vi "calibrate RP.vi"() -> ()   [LabVIEW 2018]
uses:
  Libraries/Instruments/Pulse Driver/Pusle Driver Configuration.ctl
  Libraries/Red Pitaya/RP EEPROM Calibration.ctl
  Libraries/Red Pitaya/Red Pitaya Digitizer/Red Pitaya Digitizer.lvclass
  C:/github/NHMFL_Core/Libraries/Instruments/Pulse Driver/Pulse Driver.lvclass
  Libraries/Red Pitaya/Red Pitaya Digitizer/Red Pitaya Digitizer.lvclass/Red Pitaya Digitizer.ctl
  Libraries/Red Pitaya/Red Pitaya Digitizer/Read RP Instrument.vi
  Libraries/Red Pitaya/Red Pitaya Digitizer/Write Server address.vi
  Libraries/Red Pitaya/RP Core/RP Instrument/RP Instrument.lvclass
panel:
  out "return code":i32
  out "Server  output":string
  in  "Write calib":bool
  in  "calib parameters":string
  in  "Read calib":bool
  out "Ch1 Mean (DC)":dbl
  out "Ch1 Peak to Peak":dbl
  out "Ch2 Mean (DC)":dbl
  out "Ch1 Peak to Peak":dbl
  out "RP EEPROM Calibration":T1 {"magic" format="%x"}
  in  "milliseconds to wait":u32
  out "Waveform Graph":i16[][](graph)
  in  "Server address":string="192.168.1.100"
  in  "Pulse Configuration":T2={"Pre-trigger duration"=0.01, "Post-trigger duration"=0.1, "Rate"=1000000.0, "Ranges"=[10.0], "Re-name channels"=[], "Active channels"="0:1", "External clock"=FALSE} {"Rate" format="%#_8pHz"; "Post-trigger duration" format="%#_6ps"; "Pre-trigger duration" format="%#_6ps"; "Ranges" format="%#_6pV"}
  in  "Read data":bool
  in  "stop":bool
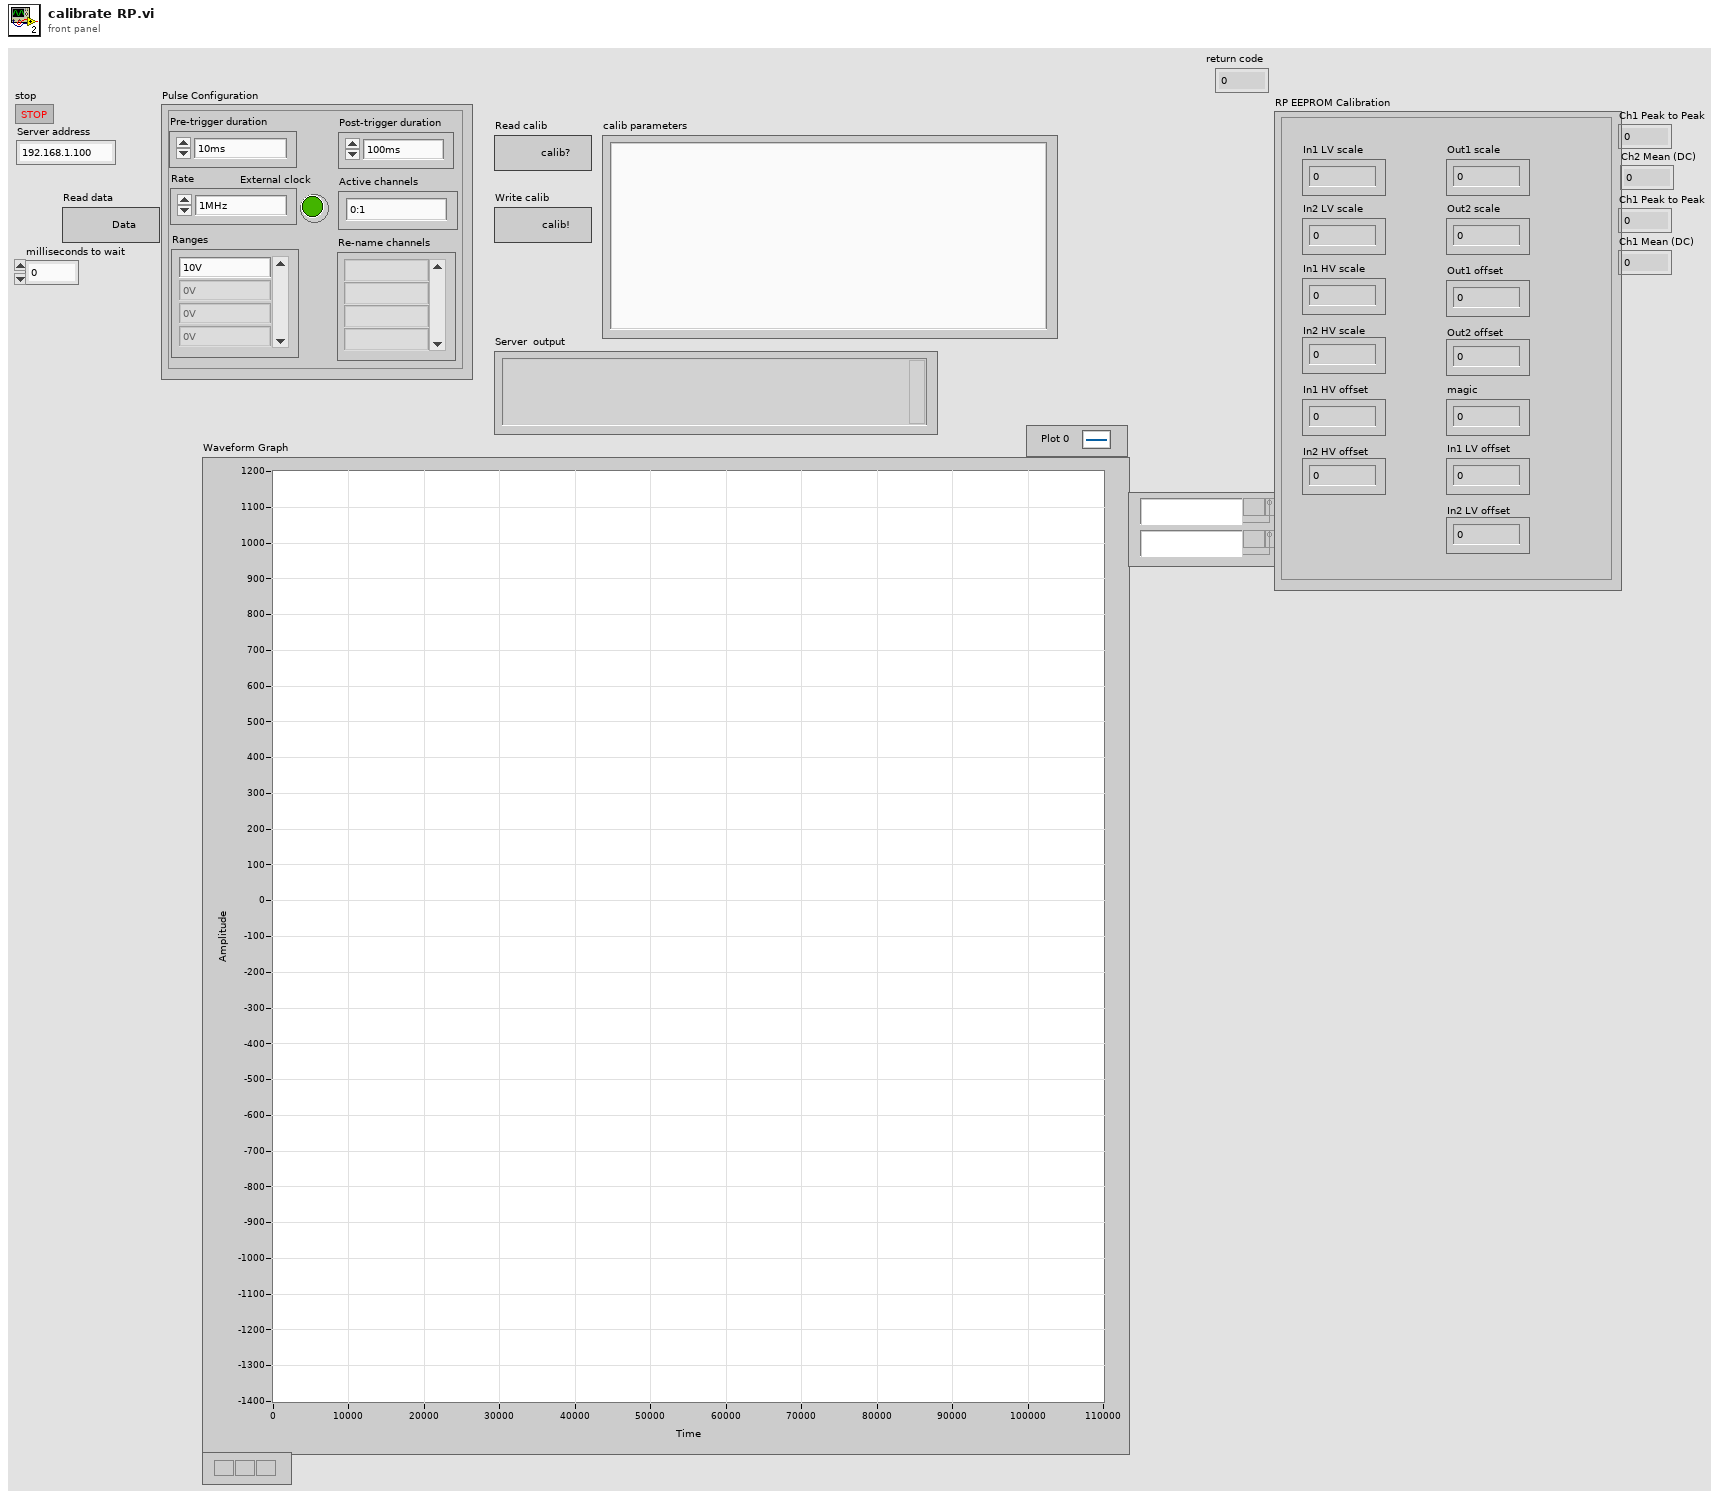
[diagram p1: front panel]
types:
  T1 = typedef "RP EEPROM Calibration.ctl" = cluster{"In1 LV scale":u32, "In2 LV scale":u32, "In1 HV scale":u32, "In2 HV scale":u32, "In1 HV offset":i32, "In2 HV offset":i32, "Out1 scale":u32, "Out2 scale":u32, "Out1 offset":i32, "Out2 offset":i32, "magic":u32, "In1 LV offset":i32, "In2 LV offset":i32}
  T2 = typedef "Pusle Driver Configuration.ctl" = cluster{"Pre-trigger duration":dbl, "Post-trigger duration":dbl, "Rate":dbl, "Ranges":dbl[], "Re-name channels":string[], "Active channels":string, "External clock":bool}
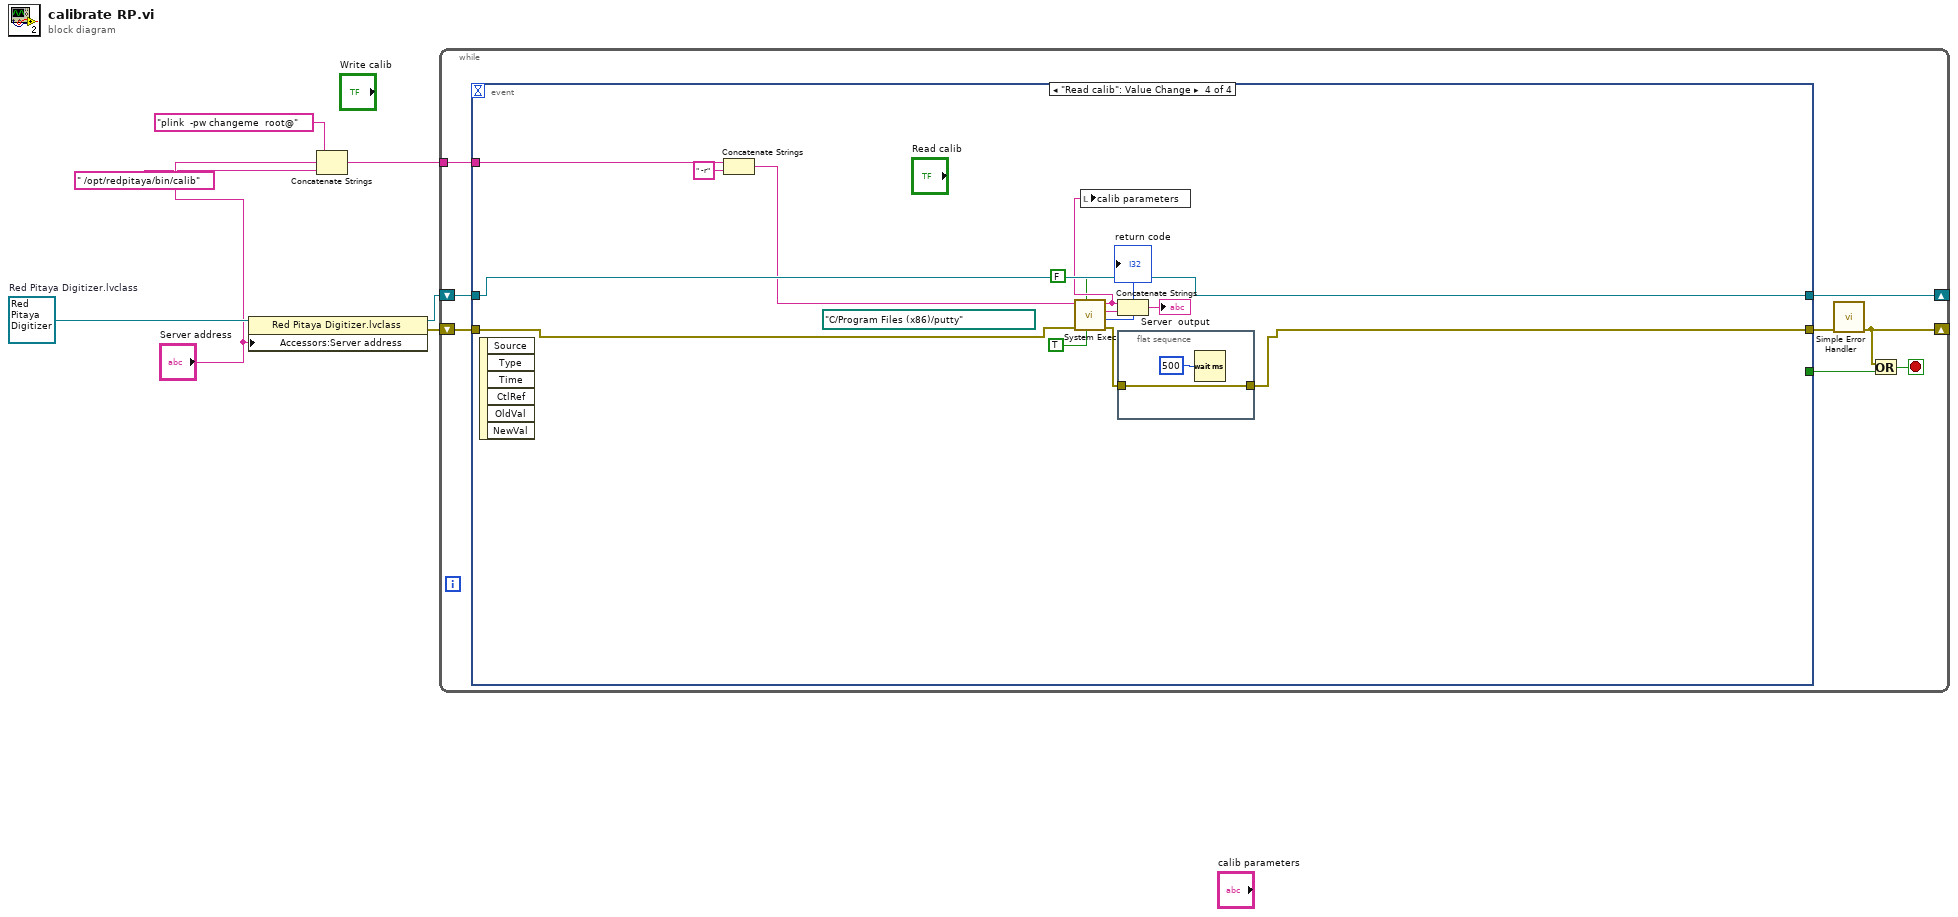
[diagram p0: block diagram]
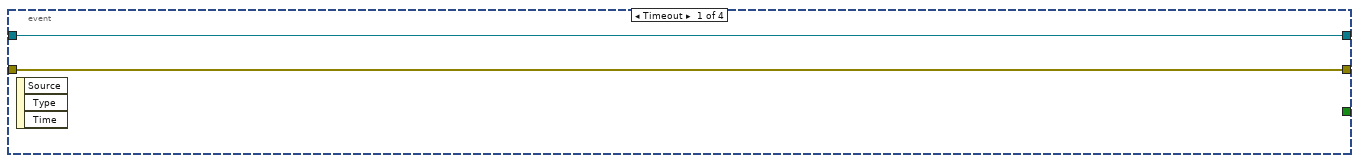
[diagram p2: hidden frame]
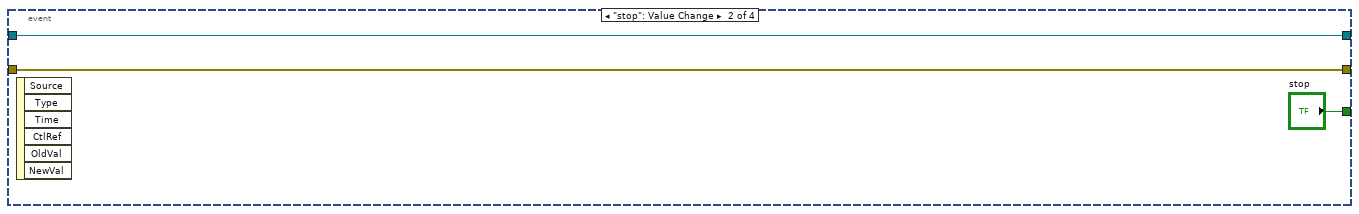
[diagram p3: hidden frame]
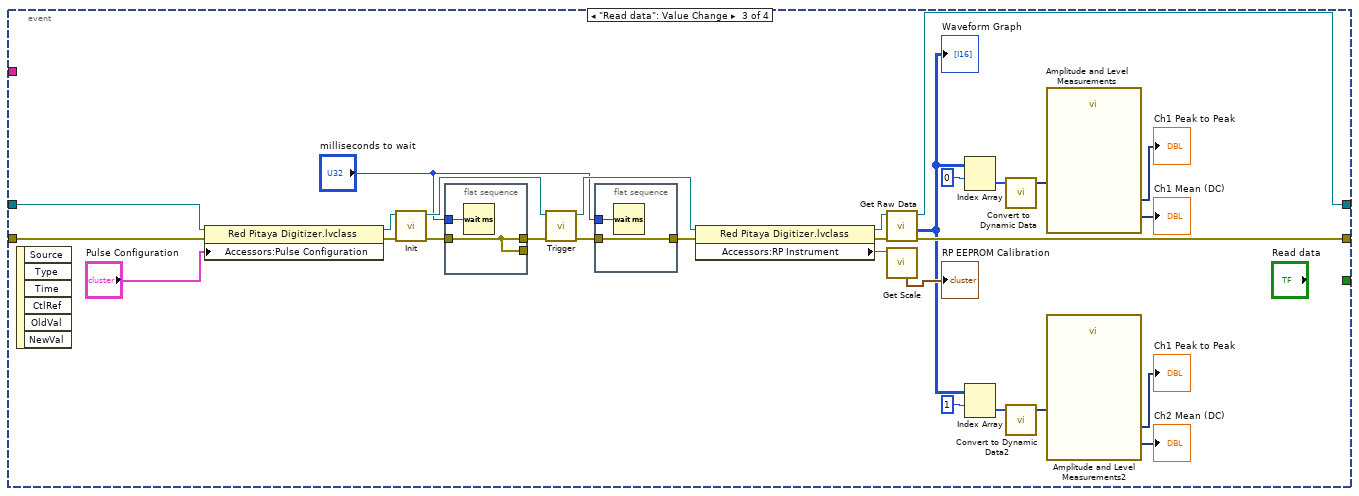
[diagram p4: hidden frame]
diagram:
  w7 = refnum<class "Red Pitaya Digitizer.lvclass"> refnum  # Red Pitaya Digitizer.lvclass
  n1 = property class="Red Pitaya Digitizer.lvclass"(reference=w7, "Accessors:Server address"="Server address") -> (reference out=w6:refnum<class "Red Pitaya Digitizer.lvclass">, error out=w5:errorcluster)  [unwired: 1 in]
  n2 = Concatenate Strings("plink  -pw changeme  root@" ("command line"), "Server address", " /opt/redpitaya/bin/calib" ("command line")) -> (w1:string)
  n3 = while {
    shift-right: [w11] -> _
    shift-left: w6 -> [w14]
    shift-right: [w9] -> _
    shift-left: w5 -> [w12]
    tunnel: w1 -> [w8]
    stop <- w10 stop-if-true
    n4 = event shown="[3] \"Read calib\": Value Change" {
      selector: _ -> [_ _ _ _]
      dyn-events: _ -> [_ _ _ _]
      timeout: _ -> [_ _ _ _]
      tunnel: [_ "stop" _ _] -> w15
      tunnel: w14 -> [w17 w19 w49 w61]
      tunnel: [w16 w18 w44 w60] -> w13
      tunnel: w12 -> [w16 w18 w43 w62]
      tunnel: [w17 w19 w42 w61] -> w11
      tunnel: w8 -> [_ _ _ w59]
      event Timeout {
        n5 = event-data() -> ()  [unwired: 1 in, 3 out]
      }
      event "stop": Value Change {
        n6 = event-data() -> ()  [unwired: 1 in, 6 out]
      }
      event "Read data": Value Change {
        n7 = event-data() -> ()  [unwired: 1 in, 6 out]
        n8 = property class="Red Pitaya Digitizer.lvclass"(reference=w49, error in=w43, "Accessors:Pulse Configuration"="Pulse Configuration") -> (reference out=w47:refnum<class "Red Pitaya Digitizer.lvclass">, error out=w45:errorcluster)
        n9 = call-dynamic "Init.vi"("error in (no error)"=w45, "Instrument Driver in"=w47) -> ("error out"=w33:errorcluster, "Instrument Driver out"=w46:refnum<class "Red Pitaya Digitizer.lvclass">)  [unwired: 7 in, 1 out]
        n10 = flat-sequence {
          tunnel: w33 -> [w50]
          tunnel: [w50] -> _
          tunnel: "milliseconds to wait" -> [w51]
          tunnel: [w50] -> w32
          frame #0 {
            n11 = Wait (ms)(milliseconds to wait=w51) -> ()  [unwired: 1 out]
          }
        }
        n12 = call-dynamic "Trigger.vi"("error in (no error)"=w32, "Red Pitaya Digitizer in"=w46) -> ("error out"=w41:errorcluster, "Red Pitaya Digitizer out"=w38:refnum<class "Red Pitaya Digitizer.lvclass">)  [unwired: 8 in]
        n13 = flat-sequence {
          tunnel: w41 -> [w53]
          tunnel: [w53] -> w40
          tunnel: "milliseconds to wait" -> [w52]
          frame #0 {
            n14 = Wait (ms)(milliseconds to wait=w52) -> ()  [unwired: 1 out]
          }
        }
        n15 = property class="Red Pitaya Digitizer.lvclass"(reference=w38, error in=w40) -> (reference out=w37:refnum<class "Red Pitaya Digitizer.lvclass">, error out=w39:errorcluster, "Accessors:RP Instrument"=w36:refnum<class "RP Instrument.lvclass">)
        n16 = call-dynamic "Get Raw Data.vi"("error in (no error)"=w39, "Red Pitaya Digitizer in"=w37) -> ("error out"=w44:errorcluster, "appended array"=w28:i16[][], "Red Pitaya Digitizer out"=w42:refnum<class "Red Pitaya Digitizer.lvclass">)  [unwired: 7 in]
        "Waveform Graph" <- w28
        n17 = call-dynamic "Get Scale.vi"("RP Instrument in"=w36) -> ("RP EEPROM Calibration"=→"RP EEPROM Calibration":T1)  [unwired: 6 in, 4 out]
        n18 = Index Array(array=w28, index (row)=0) -> (element=w30:i16[])  [unwired: 1 in]
        n19 = Index Array(array=w28, index (row)=1) -> (element=w27:i16[])  [unwired: 1 in]
        n20 = call "Convert to Dynamic Data"("Array"=w30) -> ("Dynamic Data Type"=w29:dynamicdata)  [unwired: 3 in]
        n21 = call "Convert to Dynamic Data2"("Array"=w27) -> ("Dynamic Data Type"=w26:dynamicdata)  [unwired: 3 in]
        n22 = call "Amplitude and Level Measurements"("Signals"=w29) -> ("Mean (DC)"=→"Ch1 Mean (DC)":dynamicdata, "Peak to Peak"=→"Ch1 Peak to Peak":dynamicdata)  [unwired: 12 in, 1 out]
        n23 = call "Amplitude and Level Measurements2"("Signals"=w26) -> ("Mean (DC)"=→"Ch2 Mean (DC)":dynamicdata, "Peak to Peak"=→"Ch1 Peak to Peak":dynamicdata)  [unwired: 12 in, 1 out]
      }
      event "Read calib": Value Change {
        (unwired) path "C:/Program Files (x86)/putty" ("working directory")
        n24 = event-data() -> ()  [unwired: 1 in, 6 out]
        n25 = Concatenate Strings(w59, " -r" ("string")) -> (w57:string)
        n26 = call <vilib>:"System Exec.vi"("run minimized? (F)"=TRUE, "wait until completion? (T)"=FALSE, "error in (no error)"=w62, "command line"=w57) -> ("error out"=w63:errorcluster, "return code"=→"return code":i32, "standard error"=w65:string, "standard output"=w56:string)  [unwired: 4 in]
        n27 = local write "calib parameters"(w56) -> ()
        n28 = Concatenate Strings(w56, w65) -> (→"Server  output":string)
        n29 = flat-sequence {
          tunnel: w63 -> [w68]
          tunnel: [w68] -> w60
          frame #0 {
            n30 = Wait (ms)(milliseconds to wait=u32 500) -> ()  [unwired: 1 out]
          }
        }
      }
    }
    n31 = call <vilib>:"Simple Error Handler.vi"("error in (no error)"=w13) -> ("error out"=w9:errorcluster)  [unwired: 4 in, 4 out]
    n32 = Or(x=w9, y=w15) -> (x .or. y?=w10:bool)
  }
